vi "SetParam.vi"(8 "error in (no error)":errorcluster caption="entrée d'erreur (pas d'erreur)", 10 "TfidfTransformer":T1={"norm"="l2", "use_idf"=TRUE, "smooth_idf"=TRUE, "sublinear_tf"=FALSE}, 11 "TfidfTransformer.lvclass":refnum<class "TfidfTransformer.lvclass">) -> (0 "error out":errorcluster caption="sortie d'erreur", 3 "TfidfTransformer.lvclass":refnum<class "TfidfTransformer.lvclass">)   [LabVIEW 2020, in "TfidfTransformer.lvclass"]
doc: "Set Parameters"
uses:
  TfidfTransformer.lvclass
  TfidfTransformer.lvclass/TfidfTransformer.ctl
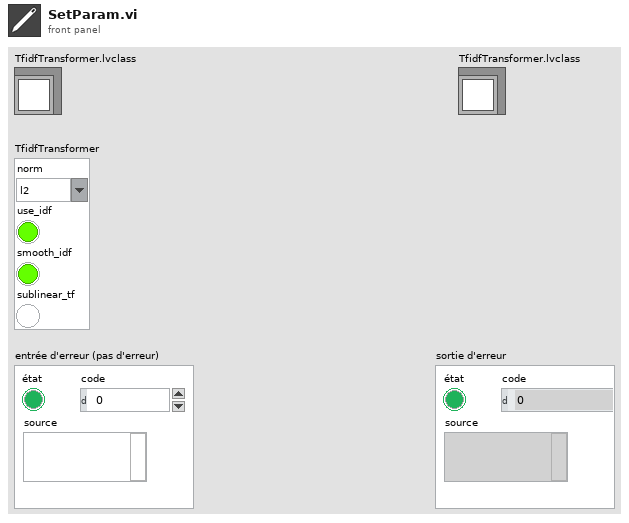
[diagram p1: front panel]
types:
  T1 = cluster{"norm":string, "use_idf":bool, "smooth_idf":bool, "sublinear_tf":bool}
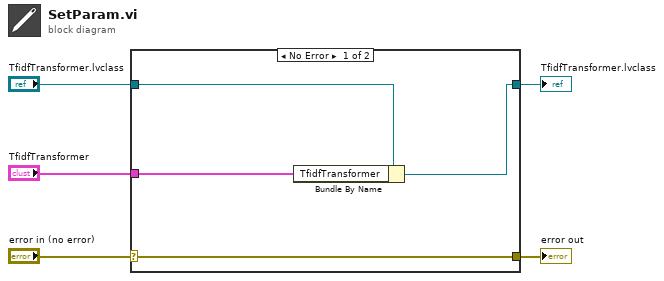
[diagram p0: block diagram]
diagram:
  n1 = case shown="No Error" "error in (no error)" {
    selector: "error in (no error)" -> [w9 w10]
    tunnel: [w9 w10] -> w4
    tunnel: [w7 w11] -> w2
    tunnel: "TfidfTransformer.lvclass" -> [w8 w11]
    tunnel: "TfidfTransformer" -> [w6 _]
    frame No Error {
      n2 = Bundle By Name(cluster=w8, "TfidfTransformer"=w6) -> (w7:refnum<class "TfidfTransformer.lvclass">)
    }
    frame Error {
    }
  }
  "error out" <- w4
  "TfidfTransformer.lvclass" <- w2
